vi "Main.vi"(8 "error in (no error)":errorcluster, 11 "TomoConversionBase in":refnum<class "TomoConversion.lvclass">) -> (0 "error out":errorcluster, 3 "component":refnum<class "TomoConversion.lvclass">)   [LabVIEW 2012, in "TomoConversion.lvclass"]
doc: "Main VI of the component."
uses:
  TomoConversion.lvclass
  small volume downsampling.ctl
  <vilib>/Distrio/Murmex/InitialiseMessage/InitialiseMessage.lvclass
  TomoConversion.lvclass/TomoConversion.ctl
  <vilib>/Distrio/Murmex/TerminateMessage/TerminateMessage.lvclass
  <vilib>/Distrio/Murmex/ConfigureMessage/ConfigureMessage.lvclass
  <vilib>/Distrio/Murmex/StopMessage/StopMessage.lvclass
  <vilib>/Distrio/Murmex/StartMessage/StartMessage.lvclass
  <vilib>/Distrio/Murmex/Murmex/update_cluster.ctl
  <vilib>/Distrio/Murmex/Murmex/Set configure at initialise.vi
  <vilib>/Distrio/Murmex/Murmex/Set log reference.vi
  <vilib>/Distrio/Murmex/Murmex/Set VI reference.vi
  <vilib>/Distrio/Murmex/Murmex/Murmex.lvclass
panel:
  in  "button::start":bool
  in  "Tab Control":enum32{"User", "Debug"}(tab)
  in  "small volume z downsampling":i32
  in  "small volume xy downsampling":T1=1 items=["2x2", "4x4", "8x8", "16x16", "32x32", "64x64"]
  in  "2x2 downsampling?":bool
  out "progress":u8 caption="conversion completed" format="%d%%"
  out "Converted cxd files":i32
  out "Number of cxd files":i32
  out "Conversion progress":u8(slide) scale=0.0..100.0
  in  "Delete original cxd files?":bool
  in  "Slices per tiff file":u32=100
  in  "ID":string="conv"
  out "log":string
  in  "button::configure":bool
  in  "button::quit":bool
  in  "terminate?":bool
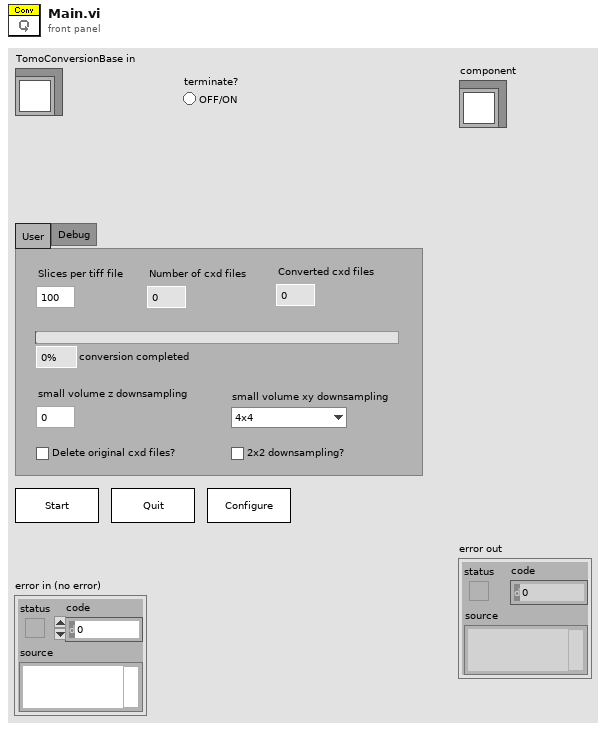
[diagram p1: front panel]
types:
  T1 = typedef "TomoConversion.lvclass/small volume downsampling.ctl" = i32
  T2 = typedef "Murmex.lvlib/Murmex.lvclass/update_cluster.ctl" = cluster{"target ID":string, "key chains":string[], "values":variant[]}
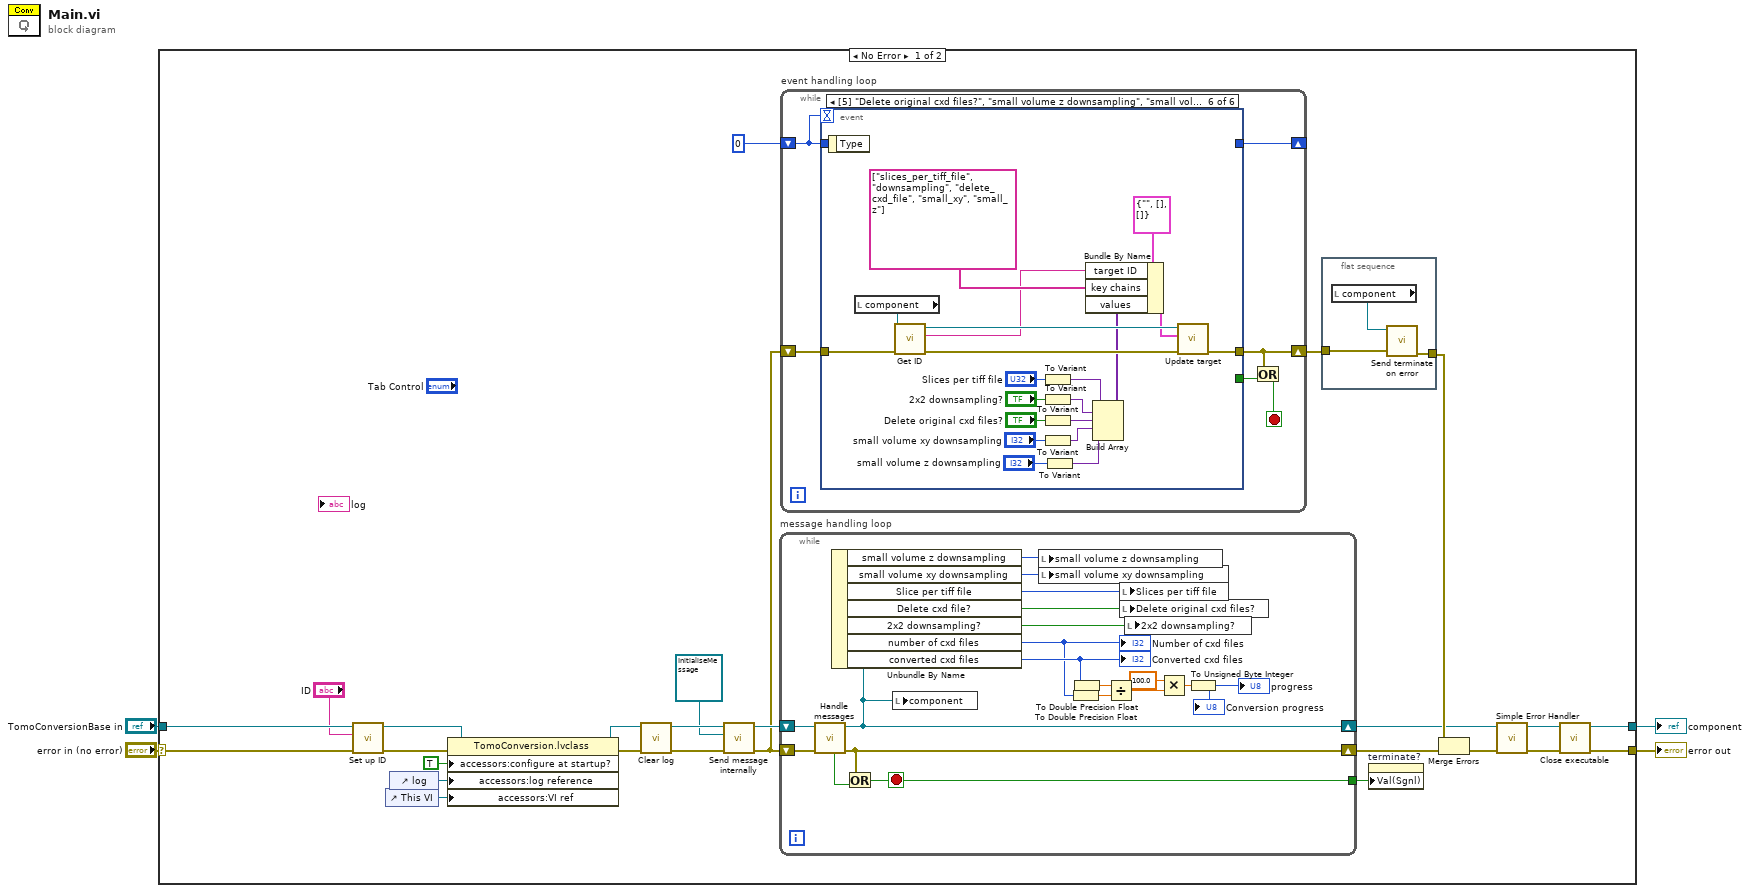
[diagram p0: block diagram]
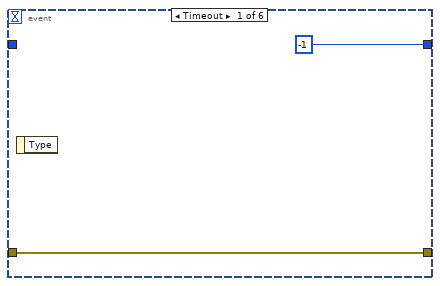
[diagram p2: hidden frame]
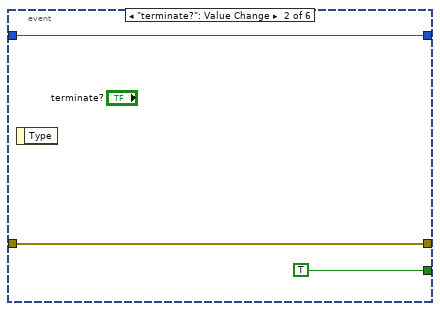
[diagram p3: hidden frame]
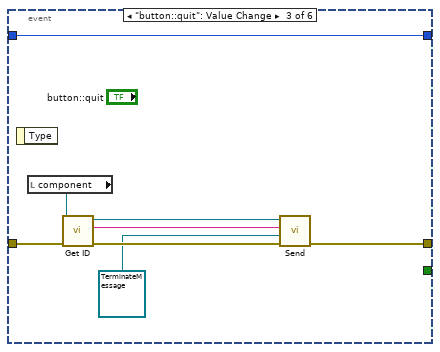
[diagram p4: hidden frame]
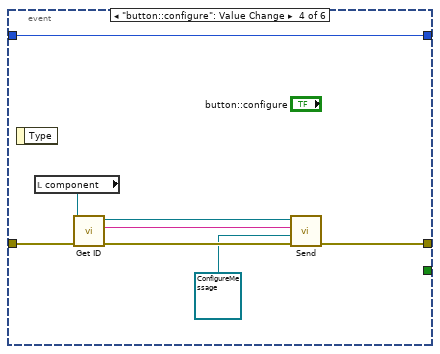
[diagram p5: hidden frame]
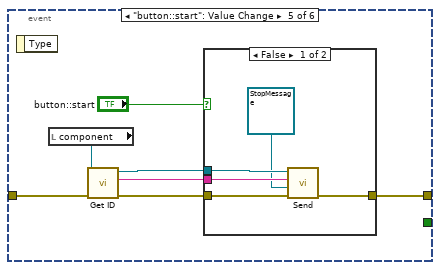
[diagram p6: hidden frame]
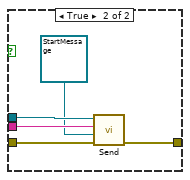
[diagram p7: hidden frame]
diagram:
  n1 = case shown="No Error" "error in (no error)" {
    selector: "error in (no error)" -> [w29 w116]
    tunnel: "TomoConversionBase in" -> [w28 w117]
    tunnel: [w5 w117] -> w2
    tunnel: [w7 w116] -> w1
    frame No Error {
      n2 = call <vilib>:"Set up ID.vi"("error in (no error)"=w29, "component ID"="ID", "MurmexBase in"=w28) -> ("error out"=w26:errorcluster, "MurmexBase out"=w25:refnum<class "TomoConversion.lvclass">)  [unwired: 6 in, 1 out]
      n3 = control-ref of="This VI"() -> (w23:refnum<vi>)
      n4 = control-ref of="log"() -> (w24:refnum<vi>)
      n5 = property class="TomoConversion.lvclass"(reference=w25, error in=w26, "accessors:configure at startup?"=TRUE ("configure at startup?"), "accessors:log reference"=w24, "accessors:VI ref"=w23) -> (reference out=w20:refnum<class "TomoConversion.lvclass">, error out=w21:errorcluster)
      n6 = call <vilib>:"Clear log.vi"("error in (no error)"=w21, "MurmexBase in"=w20) -> ("error out"=w19:errorcluster, "MurmexBase out"=w18:refnum<class "TomoConversion.lvclass">)  [unwired: 8 in]
      n7 = call <vilib>:"Send message internally.vi"("error in (no error)"=w19, "Message"=refnum<class "InitialiseMessage.lvclass"> refnum ("Distrio Murmex 1.1:InitialiseMessage"), "Murmex in"=w18) -> ("error out"=w15:errorcluster, "Murmex out"=w16:refnum<class "TomoConversion.lvclass">)  [unwired: 7 in]
      n8 = while "message handling loop" {
        shift-right: [w110] -> w6
        shift-left: w16 -> [w114]
        shift-right: [w112] -> w12
        shift-left: w15 -> [w115]
        tunnel: [w111] -> w13
        stop <- w111 stop-if-true
        n9 = call <vilib>:"Handle messages.vi"("error in (no error)"=w115, "Murmex in"=w114) -> ("error out"=w112:errorcluster, "Murmex out"=w110:refnum<class "TomoConversion.lvclass">, "terminated?"=w113:bool)  [unwired: 7 in]
        n10 = Unbundle By Name(w110) -> ("small volume z downsampling"=w97:i32, "small volume xy downsampling"=w98:T1, "Slice per tiff file"=w109:u32, "Delete cxd file?"=w107:bool, "2x2 downsampling?"=w108:bool, "number of cxd files"=w105:i32, "converted cxd files"=w106:i32)
        "Number of cxd files" <- w105
        "Converted cxd files" <- w106
        n11 = Or(x=w112, y=w113) -> (x .or. y?=w111:bool)
        n12 = local write "component"(w110) -> ()
        n13 = local write "small volume z downsampling"(w97) -> ()
        n14 = local write "small volume xy downsampling"(w98) -> ()
        n15 = To Double Precision Float(number=w105) -> (double precision float=w103:dbl)
        n16 = To Double Precision Float(number=w106) -> (double precision float=w104:dbl)
        n17 = Divide(x=w104, y=w103) -> (x/y=w102:dbl)
        n18 = local write "Slices per tiff file"(w109) -> ()
        n19 = local write "Delete original cxd files?"(w107) -> ()
        n20 = local write "2x2 downsampling?"(w108) -> ()
        n21 = Multiply(x=100.0, y=w102) -> (x*y=w101:dbl)
        n22 = To Unsigned Byte Integer(number=w101) -> (unsigned 8bit integer=→"Conversion progress" →"progress":u8)
      }
      n23 = while "event handling loop" {
        shift-right: [w37] -> _
        shift-left: 0 -> [w38]
        shift-right: [w35] -> w10
        shift-left: w15 -> [w36]
        stop <- w33 stop-if-true
        n24 = event shown="[5] \"Delete original cxd files?\", \"small volume z downsampling\", \"small volume xy downsampling\", \"Slices per tiff file\", \"2x2 downsampling?\": Value Change" {
          selector: _ -> [_ _ _ _ _ _]
          dyn-events: _ -> [_ _ _ _ _ _]
          timeout: w38 -> [_ _ _ _ _ _]
          tunnel: w38 -> [_ w42 w44 w52 _ _]
          tunnel: [-1 w42 w44 w52 _ _] -> w37
          tunnel: w36 -> [w39 w43 w51 w56 w63 w93]
          tunnel: [w39 w43 w48 w54 w62 w89] -> w35
          tunnel: [_ TRUE _ _ _ _] -> w34
          event Timeout {
            n25 = event-data() -> ()  [unwired: 1 in, 1 out]
          }
          event "terminate?": Value Change {
            n26 = event-data() -> ()  [unwired: 1 in, 1 out]
          }
          event "button::quit": Value Change {
            n27 = event-data() -> ()  [unwired: 1 in, 1 out]
            n28 = local read "component"() -> (w50:refnum<class "TomoConversion.lvclass">)
            n29 = call <vilib>:"Get ID.vi"("error in (no error)"=w51, "Murmex in"=w50) -> ("error out"=w49:errorcluster, "component id"=w46:string, "Murmex out"=w47:refnum<class "TomoConversion.lvclass">)  [unwired: 7 in]
            n30 = call <vilib>:"Send.vi"("error in (no error)"=w49, "Message"=refnum<class "TerminateMessage.lvclass"> refnum ("Distrio Murmex 1.1:TerminateMessage"), "recipient"=w46, "Murmex in"=w47) -> ("error out"=w48:errorcluster)  [unwired: 6 in, 1 out]
          }
          event "button::configure": Value Change {
            n31 = event-data() -> ()  [unwired: 1 in, 1 out]
            n32 = local read "component"() -> (w55:refnum<class "TomoConversion.lvclass">)
            n33 = call <vilib>:"Get ID.vi"("error in (no error)"=w56, "Murmex in"=w55) -> ("error out"=w59:errorcluster, "component id"=w57:string, "Murmex out"=w58:refnum<class "TomoConversion.lvclass">)  [unwired: 7 in]
            n34 = call <vilib>:"Send.vi"("error in (no error)"=w59, "Message"=refnum<class "ConfigureMessage.lvclass"> refnum ("Distrio Murmex 1.1:ConfigureMessage"), "recipient"=w57, "Murmex in"=w58) -> ("error out"=w54:errorcluster)  [unwired: 6 in, 1 out]
          }
          event "button::start": Value Change {
            n35 = event-data() -> ()  [unwired: 1 in, 1 out]
            n36 = local read "component"() -> (w61:refnum<class "TomoConversion.lvclass">)
            n37 = call <vilib>:"Get ID.vi"("error in (no error)"=w63, "Murmex in"=w61) -> ("error out"=w66:errorcluster, "component id"=w64:string, "Murmex out"=w65:refnum<class "TomoConversion.lvclass">)  [unwired: 7 in]
            n38 = case shown="False" "button::start" {
              tunnel: w66 -> [w71 w76]
              tunnel: w65 -> [w68 w75]
              tunnel: w64 -> [w69 w74]
              tunnel: [w70 w73] -> w62
              frame False {
                n39 = call <vilib>:"Send.vi"("error in (no error)"=w71, "Message"=refnum<class "StopMessage.lvclass"> refnum ("Distrio Murmex 1.2:StopMessage"), "recipient"=w69, "Murmex in"=w68) -> ("error out"=w70:errorcluster)  [unwired: 6 in, 1 out]
              }
              frame True {
                n40 = call <vilib>:"Send.vi"("error in (no error)"=w76, "Message"=refnum<class "StartMessage.lvclass"> refnum ("Distrio Murmex 1.2:StartMessage"), "recipient"=w74, "Murmex in"=w75) -> ("error out"=w73:errorcluster)  [unwired: 6 in, 1 out]
              }
            }
          }
          event "Delete original cxd files?", "small volume z downsampling", "Slices per tiff file", "2x2 downsampling?": Value Change {
            n41 = event-data() -> ()  [unwired: 1 in, 1 out]
            n42 = local read "component"() -> (w92:refnum<class "TomoConversion.lvclass">)
            n43 = call <vilib>:"Get ID.vi"("error in (no error)"=w93, "Murmex in"=w92) -> ("error out"=w88:errorcluster, "component id"=w84:string, "Murmex out"=w87:refnum<class "TomoConversion.lvclass">)  [unwired: 7 in]
            n44 = To Variant(anything="Slices per tiff file") -> (Variant=w91:variant)
            n45 = To Variant(anything="2x2 downsampling?") -> (Variant=w90:variant)
            n46 = To Variant(anything="Delete original cxd files?") -> (Variant=w79:variant)
            n47 = To Variant(anything="small volume xy downsampling") -> (Variant=w78:variant)
            n48 = To Variant(anything="small volume z downsampling") -> (Variant=w77:variant)
            n49 = Build Array(w91, w90, w79, w78, w77) -> (w85:variant[])
            n50 = Bundle By Name(cluster=T2 {"target ID"="", "key chains"=[], "values"=[]} ("update cluster"), "target ID"=w84, "key chains"=string[] ["slices_per_tiff_file", "downsampling", "delete_cxd_file", "small_xy", "small_z"], "values"=w85) -> (w86:T2)
            n51 = call <vilib>:"Update target.vi"("error in (no error)"=w88, "update cluster"=w86, "MurmexBase in"=w87) -> ("error out"=w89:errorcluster)  [unwired: 7 in, 1 out]
          }
        }
        n52 = Or(x=w35, y=w34) -> (x .or. y?=w33:bool)
      }
      n53 = flat-sequence {
        tunnel: w10 -> [w32]
        tunnel: [w31] -> w9
        frame #0 {
          n54 = local read "component"() -> (w30:refnum<class "TomoConversion.lvclass">)
          n55 = call <vilib>:"Send terminate on error.vi"("error in (no error)"=w32, "Murmex in"=w30) -> ("error out"=w31:errorcluster)  [unwired: 8 in, 1 out]
        }
      }
      n56 = property on="terminate?" class="Bool (strict)"("Val(Sgnl)"=w13) -> ()  [unwired: 2 in, 2 out]
      n57 = Merge Errors(w9, w12) -> (w11:errorcluster)
      n58 = call <vilib>:"Simple Error Handler.vi"("error in (no error)"=w11) -> ("error out"=w8:errorcluster)  [unwired: 4 in, 4 out]
      n59 = call <vilib>:"Close executable.vi"("error in (no error)"=w8, "MurmexBase in"=w6) -> ("error out"=w7:errorcluster, "MurmexBase out"=w5:refnum<class "TomoConversion.lvclass">)  [unwired: 8 in]
    }
    frame Error {
    }
  }
  "error out" <- w1
  "component" <- w2
